vi "close.vi"(8 "error in (no error)":errorcluster, 11 "OHAUS AV8101 in":refnum<class "OHAUS AV8101.lvclass">) -> (0 "error out":errorcluster, 3 "OHAUS AV8101 out":refnum<class "OHAUS AV8101.lvclass">)   [LabVIEW 2015, in "OHAUS AV8101.lvclass"]
uses:
  OHAUS AV8101.lvclass
  OHAUS AV8101.lvclass/OHAUS AV8101.ctl
  OHAUS AV8101 Drivers/Ohaus AV Series.lvlib
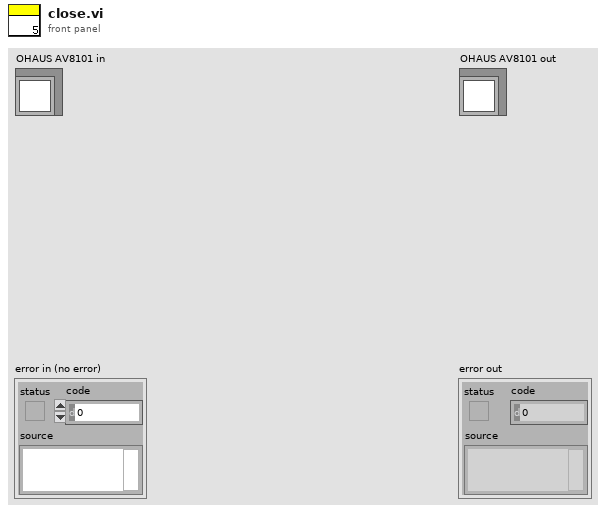
[diagram p1: front panel]
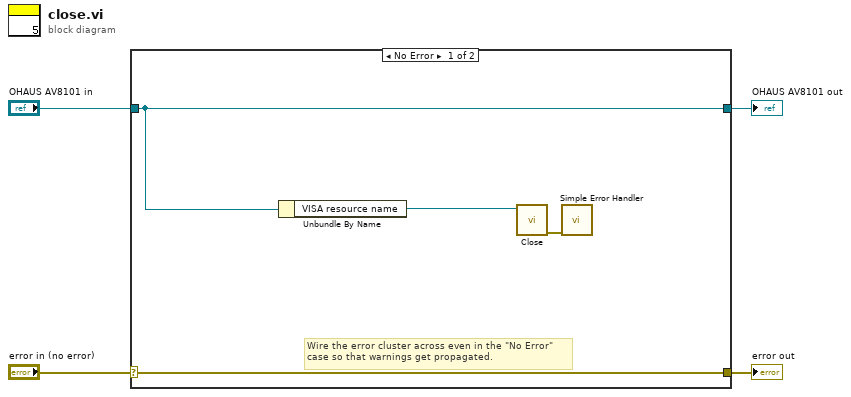
[diagram p0: block diagram]
diagram:
  n1 = case shown="No Error" "error in (no error)" {
    selector: "error in (no error)" -> [w8 w10]
    tunnel: [w8 w10] -> w3
    tunnel: [w6 w9] -> w1
    tunnel: "OHAUS AV8101 in" -> [w6 w9]
    frame No Error {
      # "Wire the error cluster across even in the \"No Error\"\ncase so that warnings get propagated."
      n2 = Unbundle By Name(w6) -> ("VISA resource name"=w5:refnum<visa-resource-name>)
      n3 = call "Close.vi"("VISA resource name"=w5) -> ("error out"=w7:errorcluster)  [unwired: 10 in]
      n4 = call <vilib>:"Simple Error Handler.vi"("error in (no error)"=w7) -> ()  [unwired: 4 in, 5 out]
    }
    frame Error {
    }
  }
  "error out" <- w3
  "OHAUS AV8101 out" <- w1
